vi "dummy.vi"() -> ()   [LabVIEW 2011]
panel:
  out "appended path":path
  out "path":path
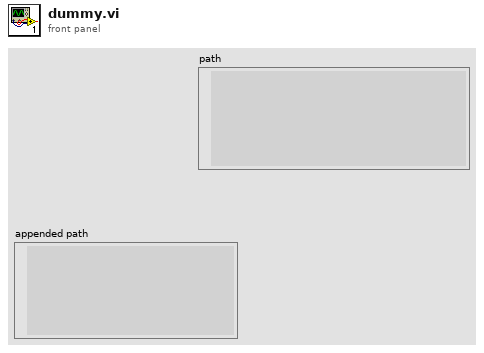
[diagram p1: front panel]
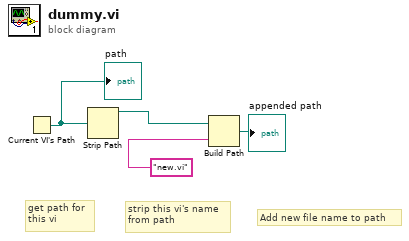
[diagram p0: block diagram]
diagram:
  # "Add new file name to path"
  # "strip this vi's name \nfrom path"
  # "get path for \nthis vi"
  n1 = Current VI's Path() -> (path=w2:path)
  "path" <- w2
  n2 = Strip Path(path=w2) -> (stripped path=w1:path)  [unwired: 1 out]
  n3 = Build Path(base path=w1, name or relative path="new.vi") -> (appended path=→"appended path":path)
